vi "createTaskStack.vi"(8 "error in (no error)":errorcluster, 11 "BuildWorker in":refnum<class "BuildWorker.lvclass">) -> (0 "error out":errorcluster, 3 "BuildWorker out":refnum<class "BuildWorker.lvclass">)   [LabVIEW 2017, in "BuildWorker.lvlib" / "BuildWorker.lvclass"]
uses:
  BuildWorker.lvclass
  Classes/Task/Task.lvclass
  BuildWorker.lvclass/BuildWorker.ctl
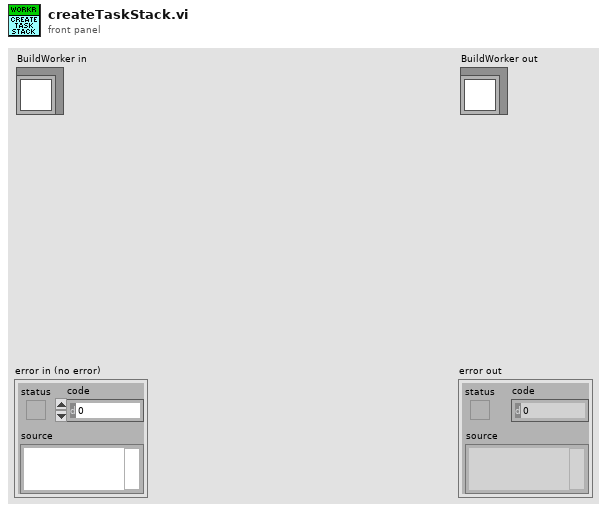
[diagram p1: front panel]
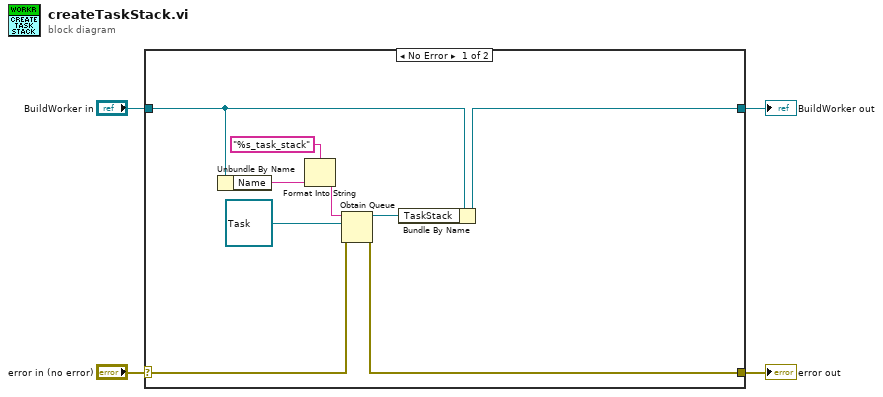
[diagram p0: block diagram]
diagram:
  n1 = case shown="No Error" "error in (no error)" {
    selector: "error in (no error)" -> [w12 w15]
    tunnel: [w11 w15] -> w3
    tunnel: [w6 w14] -> w1
    tunnel: "BuildWorker in" -> [w10 w14]
    frame No Error {
      n2 = Unbundle By Name(w10) -> ("Name"=w9:string)
      n3 = Format Into String(format string="%s_task_stack", w9) -> (resulting string=w8:string)  [unwired: 2 in, 1 out]
      n4 = Obtain Queue(name (unnamed)=w8, element data type=refnum<class "Task.lvclass"> refnum ("Task.lvclass"), error in (no error)=w12) -> (queue out=w5:refnum<queue>, error out=w11:errorcluster)  [unwired: 2 in, 1 out]
      n5 = Bundle By Name(cluster=w10, "TaskStack"=w5) -> (w6:refnum<class "BuildWorker.lvclass">)
    }
    frame Error {
    }
  }
  "error out" <- w3
  "BuildWorker out" <- w1
